vi "add Test.vi"(8 "error in (no error)":errorcluster caption="Fehler (Eingang, kein Fehler)", 10 "Test.lvclass":refnum<class "Test.lvclass">, 11 "Report (Eingang)":refnum<class "Report.lvclass">) -> (0 "error out":errorcluster caption="Fehler (Ausgang)", 3 "Report (Ausgang)":refnum<class "Report.lvclass">)   [LabVIEW 2013, in "DatenKlassen.lvlib" / "Report.lvclass"]
uses:
  Report.lvclass
  Test/Test.lvclass
  Report.lvclass/Report.ctl
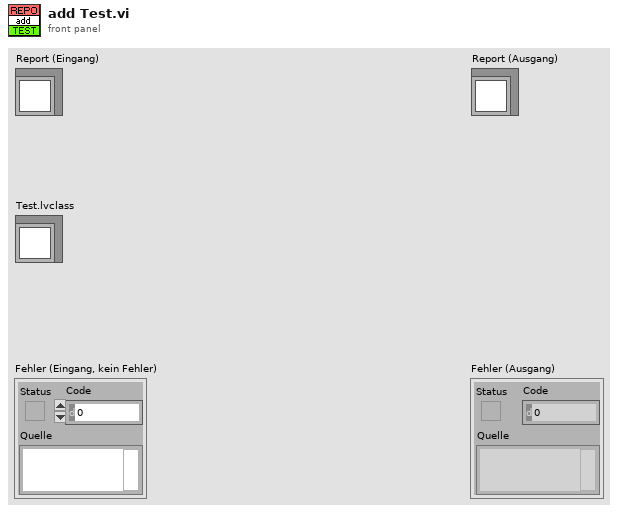
[diagram p1: front panel]
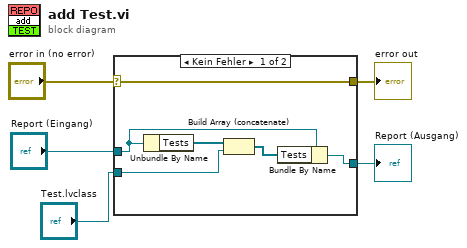
[diagram p0: block diagram]
diagram:
  n1 = case shown="Kein Fehler" "error in (no error)" {
    selector: "error in (no error)" -> [w11 w12]
    tunnel: [w11 w12] -> w4
    tunnel: [w10 w13] -> w2
    tunnel: "Report (Eingang)" -> [w9 w13]
    tunnel: "Test.lvclass" -> [w6 _]
    frame No Error {
      n2 = Unbundle By Name(w9) -> ("Tests"=w7:refnum<class "Test.lvclass">[])
      n3 = Build Array (concatenate)(w7, w6) -> (w8:refnum<class "Test.lvclass">[])
      n4 = Bundle By Name(cluster=w9, "Tests"=w8) -> (w10:refnum<class "Report.lvclass">)
    }
    frame Error {
    }
  }
  "error out" <- w4
  "Report (Ausgang)" <- w2
